vi "GA_Mutate.vi"(6 "Parameters":T1={"Population size"=100, "Generations no."=500, "Significant digits"=4, "Crossover probabality"=0.85, "Mutation mode"=enum."one-point, fixed rate", "Use Gray code?"=FALSE, "Mutation rate"=0.05, "Min mutation rate"=0.0005, "Max mutation rate"=0.25, "Reproduction plan"=enum."Steady-state-replace-worst", "Elitism"=FALSE, "Fmax"=1} {"Max mutation rate" min=0.0 max=1.0; "Min mutation rate" min=0.0 max=1.0; "Mutation rate" min=0.0 max=1.0; "Crossover probabality" min=0.0 max=1.0; "Significant digits" min=1; "Generations no." min=1; "Population size" min=1}, 11 "Genotype in":i8[](array[numeric])) -> (3 "Genotype out":i8[](array[numeric]))   [LabVIEW 2016, in "Optimal Frequency Bands Search.lvlib" / "GeneticAlgorithm.lvlib"]
doc: "Применить оператор мутации к генотипу особи"
uses:
  GeneticAlgorithm.lvlib
  GA_tParameters.ctl
panel:
  # "This VI is a part of BCI Design library, http://www.ru-bci.org \nCopyright © 2020, Sotnikov Peter, All rights reserved. License: CC BY-NC 4.0"
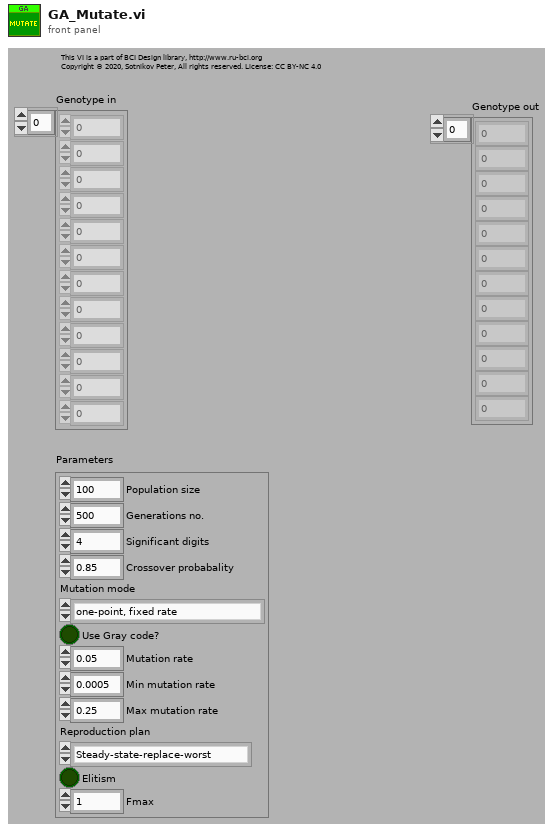
[diagram p1: front panel]
types:
  T1 = typedef "Optimal Frequency Bands Search.lvlib/GeneticAlgorithm.lvlib/GA_tParameters.ctl" = cluster{"Population size":i32, "Generations no.":i32, "Significant digits":i32, "Crossover probabality":dbl, "Mutation mode":enum16{"one-point, fixed rate", "one-point, fitness-adjustable rate", "one-point, distance-adjustable rate"}, "Use Gray code?":bool, "Mutation rate":dbl, "Min mutation rate":dbl, "Max mutation rate":dbl, "Reproduction plan":enum16{"Full generational replacement", "Steady-state-replace-random", "Steady-state-replace-worst"}, "Elitism":bool, "Fmax":i32}
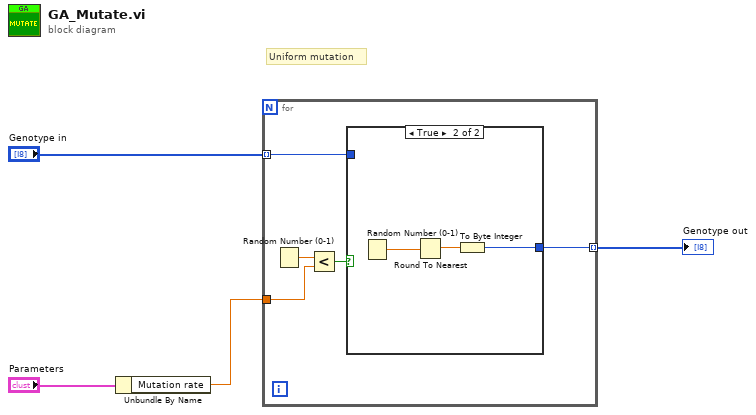
[diagram p0: block diagram]
diagram:
  # "Uniform mutation"
  n1 = Unbundle By Name("Parameters") -> ("Mutation rate"=w1:dbl)
  n2 = for {
    tunnel: "Genotype in" -> [w6] mode=indexing
    tunnel: w1 -> [w8]
    tunnel: [w5] -> w2 mode=indexing
    n3 = Random Number (0-1)() -> (number: 0 to 1=w9:dbl)
    n4 = Less?(x=w9, y=w8) -> (x < y?=w7:bool)
    n5 = case shown="True" w7 {
      tunnel: w6 -> [w10 _]
      tunnel: [w10 w12] -> w5
      frame False {
      }
      frame True {
        n6 = Random Number (0-1)() -> (number: 0 to 1=w11:dbl)
        n7 = Round To Nearest(number=w11) -> (nearest integer value=w13:dbl)
        n8 = To Byte Integer(number=w13) -> (8bit integer=w12:i8)
      }
    }
  }
  "Genotype out" <- w2
